vi "get_period.vi"(10 "period":i32, 11 "sample rate (S/s)":dbl) -> (3 "sample rate per period":dbl)   [LabVIEW 2022 SP3]
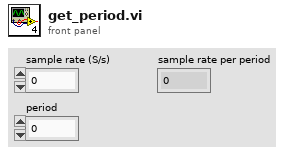
[diagram p1: front panel]
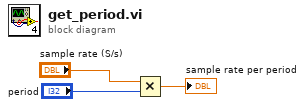
[diagram p0: block diagram]
diagram:
  n1 = Multiply(x="sample rate (S/s)", y="period") -> (x*y=→"sample rate per period":dbl)
